vi "S2C_VAR_AddVariable.vi"(8 "Error In":errorcluster, 9 "TreeRef":refnum<vi>, 10 "Array?":bool, 11 "Type":string(combo)) -> (0 "Error Out":errorcluster)   [LabVIEW 2015]
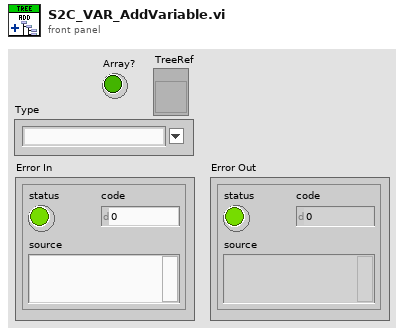
[diagram p1: front panel]
types:
  T1 = cluster{"Left Cell String":string, "Child Text":string[], "Child Tag":string, "Item Indent":i32, "Child Only?":bool, "Glyph Index":i32}[]
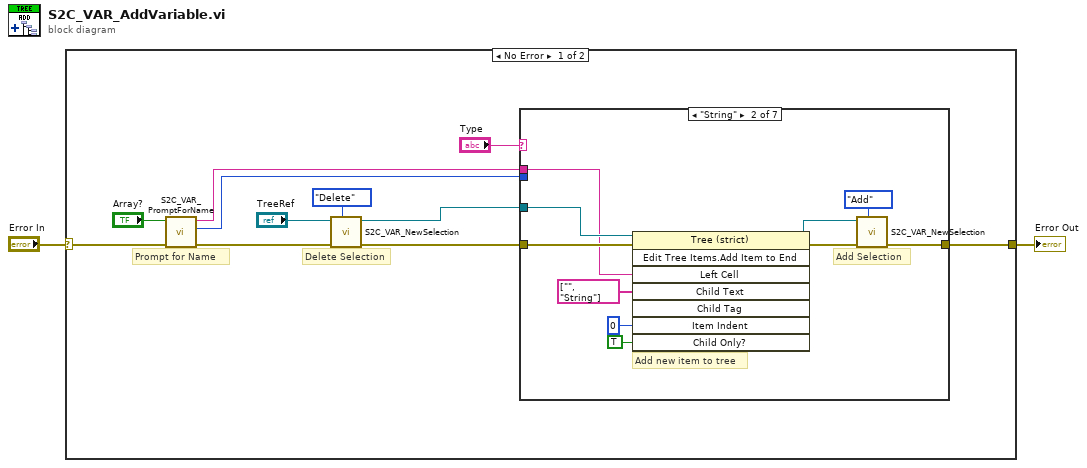
[diagram p0: block diagram]
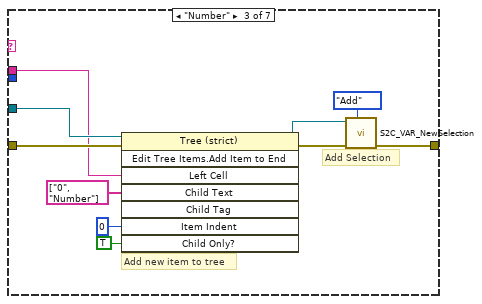
[diagram p3: hidden frame]
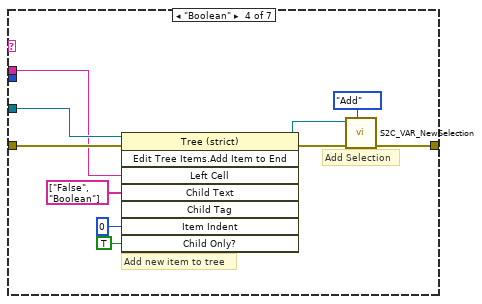
[diagram p4: hidden frame]
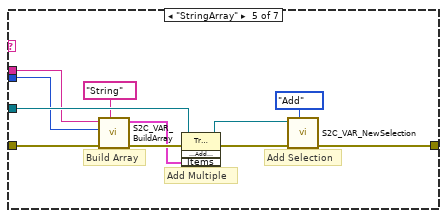
[diagram p5: hidden frame]
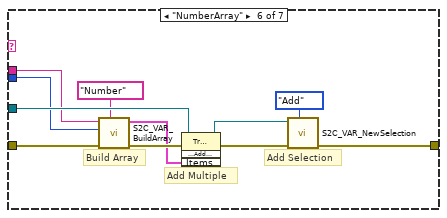
[diagram p6: hidden frame]
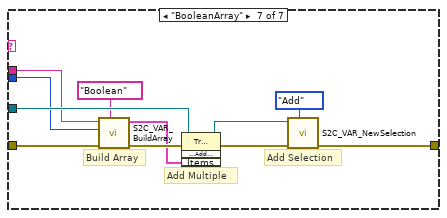
[diagram p7: hidden frame]
diagram:
  n1 = case shown="No Error" "Error In" {
    selector: "Error In" -> [w7 w78]
    tunnel: [w12 w78] -> w1
    frame No Error {
      # "Prompt for Name"
      # "Delete Selection"
      n2 = call "S2C_VAR_PromptForName.vi"("Error In"=w7, "Array?"="Array?") -> ("Error Out"=w6:errorcluster, "Size"=w4:i32, "Name"=w5:string)  [unwired: 7 in]
      n3 = call "S2C_VAR_NewSelection.vi"("Action"=enum16{"Add", "Delete"}."Delete", "Error In"=w6, "Ref In"="TreeRef") -> ("Error Out"=w11:errorcluster, "Ref Out"=w8:refnum<vi>)  [unwired: 7 in]
      n4 = case shown="\"String\"" "Type" {
        tunnel: w11 -> [w14 w24 w34 w44 w50 w61 w72]
        tunnel: w8 -> [_ w23 w33 w43 w55 w66 w77]
        tunnel: [w14 w16 w26 w36 w51 w62 w73] -> w12
        tunnel: w4 -> [_ _ _ _ w46 w57 w68]
        tunnel: w5 -> [_ w20 w30 w40 w47 w58 w69]
        frame "Other", Default {
        }
        frame "String" {
          # "Add Selection"
          # "Add new item to tree"
          n5 = invoke class="Tree (strict)" method="Edit Tree Items.Add Item to End"(reference=w23, error in=w24, "Left Cell"=w20, "Child Text"=string[] ["", "String"] ("Array"), "Item Indent"=0 ("New Item Indentation"), "Child Only?"=TRUE) -> (reference out=w18:refnum<vi>, error out=w17:errorcluster)  [unwired: 2 in, 6 out]
          n6 = call "S2C_VAR_NewSelection.vi"("Action"=enum16{"Add", "Delete"}."Add", "Error In"=w17, "Ref In"=w18) -> ("Error Out"=w16:errorcluster)  [unwired: 7 in, 1 out]
        }
        frame "Number" {
          # "Add Selection"
          # "Add new item to tree"
          n7 = invoke class="Tree (strict)" method="Edit Tree Items.Add Item to End"(reference=w33, error in=w34, "Left Cell"=w30, "Child Text"=string[] ["0", "Number"] ("Array"), "Item Indent"=0 ("New Item Indentation"), "Child Only?"=TRUE) -> (reference out=w28:refnum<vi>, error out=w27:errorcluster)  [unwired: 2 in, 6 out]
          n8 = call "S2C_VAR_NewSelection.vi"("Action"=enum16{"Add", "Delete"}."Add", "Error In"=w27, "Ref In"=w28) -> ("Error Out"=w26:errorcluster)  [unwired: 7 in, 1 out]
        }
        frame "Boolean" {
          # "Add Selection"
          # "Add new item to tree"
          n9 = invoke class="Tree (strict)" method="Edit Tree Items.Add Item to End"(reference=w43, error in=w44, "Left Cell"=w40, "Child Text"=string[] ["False", "Boolean"] ("Array"), "Item Indent"=0 ("New Item Indentation"), "Child Only?"=TRUE) -> (reference out=w38:refnum<vi>, error out=w37:errorcluster)  [unwired: 2 in, 6 out]
          n10 = call "S2C_VAR_NewSelection.vi"("Action"=enum16{"Add", "Delete"}."Add", "Error In"=w37, "Ref In"=w38) -> ("Error Out"=w36:errorcluster)  [unwired: 7 in, 1 out]
        }
        frame "StringArray" {
          # "Build Array"
          # "Add Selection"
          # "Add Multiple"
          n11 = call "S2C_VAR_BuildArray.vi"("Type"="String", "Error In"=w50, "Size"=w46, "Name"=w47) -> ("Error Out"=w48:errorcluster, "Array"=w45:T1)  [unwired: 6 in]
          n12 = invoke class="Tree (strict)" method="Edit Tree Items.Add Multiple Items to End"(reference=w55, error in=w48, "Items"=w45) -> (reference out=w52:refnum<vi>, error out=w53:errorcluster)  [unwired: 1 in, 2 out]
          n13 = call "S2C_VAR_NewSelection.vi"("Action"=enum16{"Add", "Delete"}."Add", "Error In"=w53, "Ref In"=w52) -> ("Error Out"=w51:errorcluster)  [unwired: 7 in, 1 out]
        }
        frame "NumberArray" {
          # "Build Array"
          # "Add Selection"
          # "Add Multiple"
          n14 = call "S2C_VAR_BuildArray.vi"("Type"="Number", "Error In"=w61, "Size"=w57, "Name"=w58) -> ("Error Out"=w59:errorcluster, "Array"=w56:T1)  [unwired: 6 in]
          n15 = invoke class="Tree (strict)" method="Edit Tree Items.Add Multiple Items to End"(reference=w66, error in=w59, "Items"=w56) -> (reference out=w63:refnum<vi>, error out=w64:errorcluster)  [unwired: 1 in, 2 out]
          n16 = call "S2C_VAR_NewSelection.vi"("Action"=enum16{"Add", "Delete"}."Add", "Error In"=w64, "Ref In"=w63) -> ("Error Out"=w62:errorcluster)  [unwired: 7 in, 1 out]
        }
        frame "BooleanArray" {
          # "Build Array"
          # "Add Selection"
          # "Add Multiple"
          n17 = call "S2C_VAR_BuildArray.vi"("Type"="Boolean", "Error In"=w72, "Size"=w68, "Name"=w69) -> ("Error Out"=w70:errorcluster, "Array"=w67:T1)  [unwired: 6 in]
          n18 = invoke class="Tree (strict)" method="Edit Tree Items.Add Multiple Items to End"(reference=w77, error in=w70, "Items"=w67) -> (reference out=w74:refnum<vi>, error out=w75:errorcluster)  [unwired: 1 in, 2 out]
          n19 = call "S2C_VAR_NewSelection.vi"("Action"=enum16{"Add", "Delete"}."Add", "Error In"=w75, "Ref In"=w74) -> ("Error Out"=w73:errorcluster)  [unwired: 7 in, 1 out]
        }
      }
    }
    frame Error {
    }
  }
  "Error Out" <- w1
